vi "Digital Read 1 Channel.vi"(8 "error in (no error)":errorcluster, 10 "Read":i32, 11 "Arduino in":refnum<class "Arduino.lvclass">) -> (0 "error out":errorcluster, 2 "Value":bool=TRUE, 3 "Arduino out":refnum<class "Arduino.lvclass">)   [LabVIEW 2016, in "Arduino.lvclass"]
uses:
  Arduino.lvclass
  Arduino.lvclass/Arduino.ctl
  <vilib>/MakerHub/LINX/Public/Peripherals/Digital/Digital Read 1 Chan.vi
  <vilib>/MakerHub/LINX/Public/Peripherals/Digital/Digital Read N Chans.vi
  <vilib>/MakerHub/LINX/Private/Local IO/LinxDigitalRead.vi
  <vilib>/MakerHub/LINX/Public/Utilities/Check Channel.vi
  <vilib>/MakerHub/LINX/Private/Utilties/Generate Error.vi
  <vilib>/MakerHub/LINX/LMH-LINX.lvlib
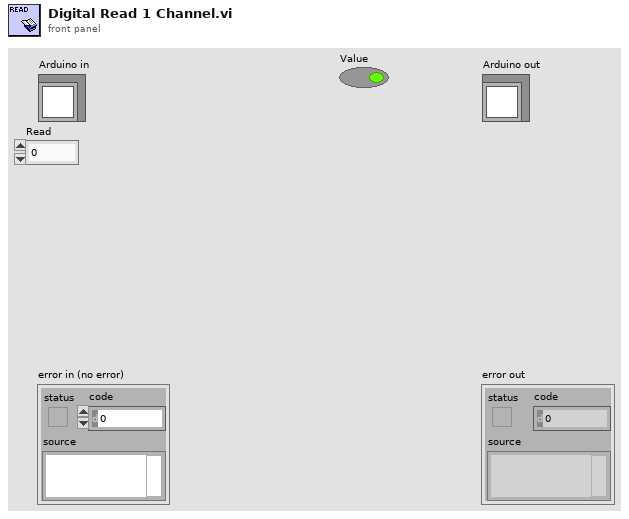
[diagram p1: front panel]
types:
  T1 = typedef "LMH-LINX.lvlib/LINX Ref.ctl" = cluster{"IO":T2, "Interface":T3, "LINX Device Config":T4}
  T2 = typedef "LMH-LINX.lvlib/Platform.ctl" = enum16{"Remote", "Local"}
  T3 = typedef "LMH-LINX.lvlib/Interface.ctl" = enum16{"Serial", "TCP"}
  T4 = typedef "LMH-LINX.lvlib/Device.lvlib/LINX Device Config.ctl" = cluster{"Interface":T3, "COM Port":refnum<visa-resource-name>, "TCP Configuration":T5, "Device Family":u8, "Device ID":u8, "Device Name":string, "TCP Ref":refnum<k5>, "Channels":T6}
  T5 = typedef "LMH-LINX.lvlib/Device.lvlib/TCP Config.ctl" = cluster{"IP Address":string, "Port":u16}
  T6 = typedef "LMH-LINX.lvlib/Channels.ctl" = cluster{"DI":u8[], "DO":u8[], "AI":u8[], "AO":u8[], "PWM":u8[], "QE":u8[], "UART":u8[], "I2C 2":u8[], "SPI":u8[], "CAN":u8[], "Servo":u8[], "AI Ref (V)":dbl, "AI Resolution (Bits)":u8, "AO Ref (V)":dbl, "AO Resolution (Bits)":u8}
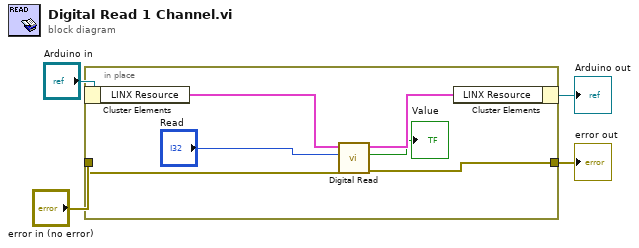
[diagram p0: block diagram]
diagram:
  n1 = in-place {
    in-place-border: "error in (no error)" -> [w6]
    in-place-border: [w5] -> w1
    n2 = in-place-cluster #1("Arduino in") -> ("LINX Resource"=w9:T1)
    n3 = call-poly <vilib>:"Digital Read.vi"("Error In"=w6, "DI Channel"="Read", "LINX Resource"=w9) -> ("Error Out"=w5:errorcluster, "DI Value"=→"Value":bool, "LINX Resource"=w8:T1)  [unwired: 6 in]
    n4 = in-place-cluster #1("LINX Resource"=w8) -> (→"Arduino out":refnum<class "Arduino.lvclass">)
  }
  "error out" <- w1
